vi "Calibration.vi"(8 "error in (no error)":errorcluster, 11 "VISA resource name In":T1={"Conection Data"="COM4"}) -> (0 "error out":errorcluster, 3 "VISA resource name Out":T1={"Conection Data"="COM4"})   [LabVIEW 2014, in "AD4212C Lib.lvlib"]
doc: "VI de calibración que se utiliza para poner a punto la balanza."
uses:
  AD4212C Lib.lvlib
  Typedef/Connection Data.ctl
  Typedef/Calibration Enum.ctl
panel:
  out "Indicator Med":string
  in  "Stop":bool
  out "Progress Bar":u64(slide) scale=0.0..6.0
  out "Indicator":string
  in  "Next":bool
  in  "Start":bool
  # "BALANCE CALIBRATION"
  # "Progress Bar"
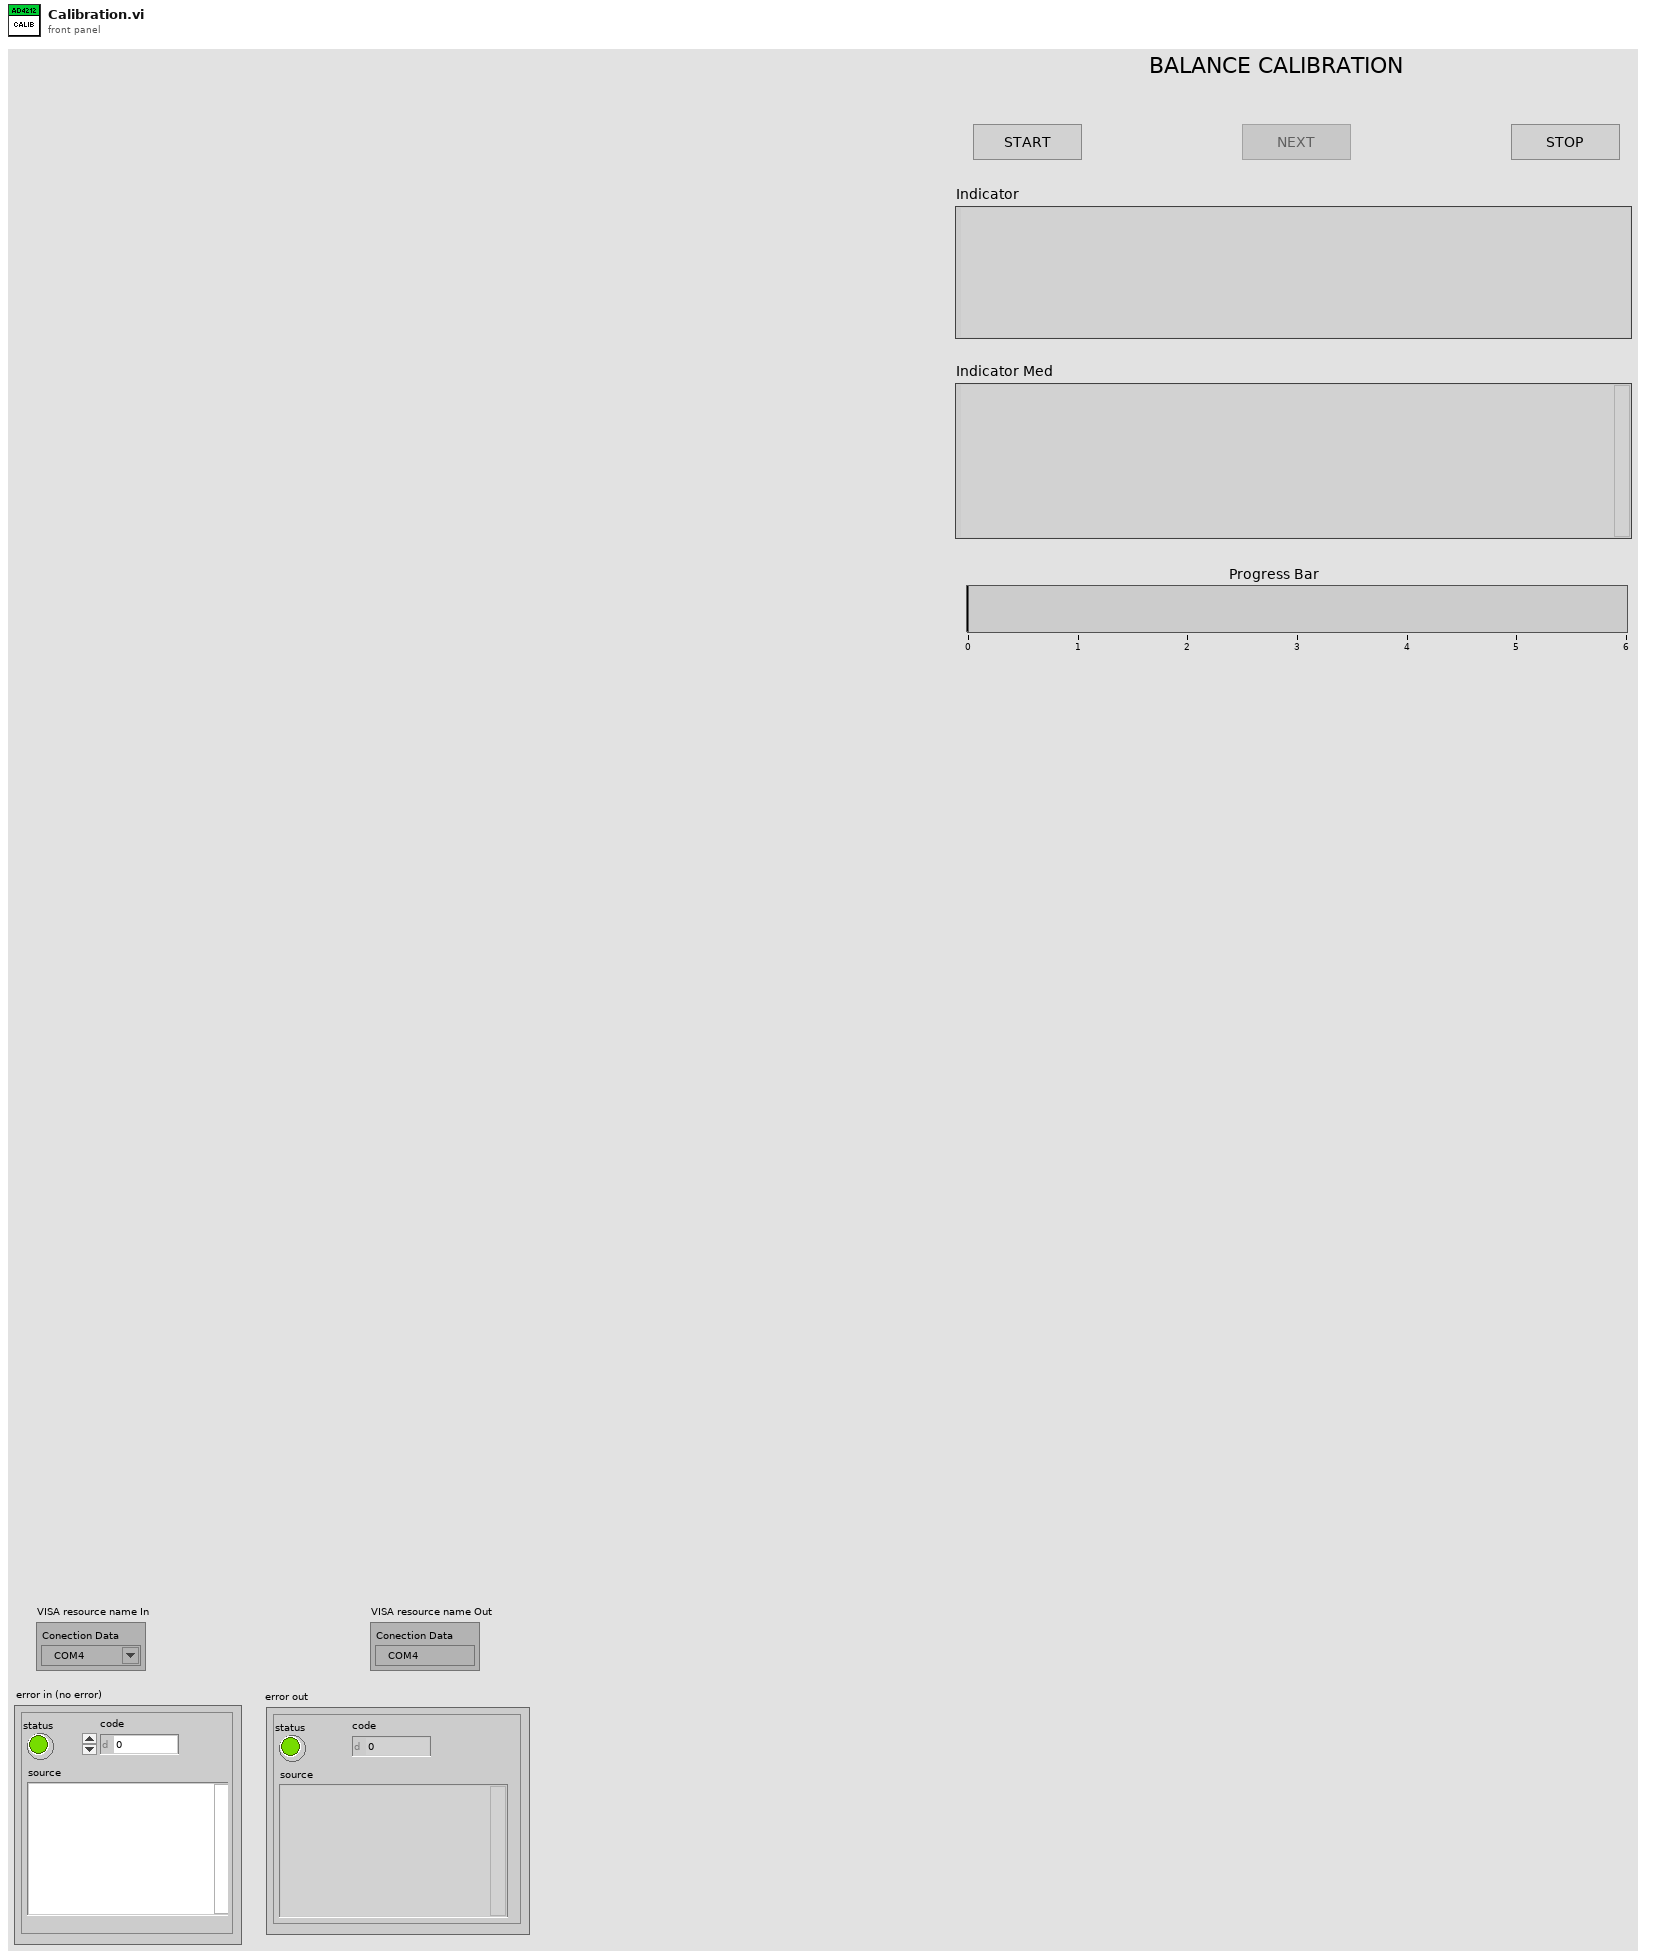
[diagram p1: front panel]
types:
  T1 = typedef "AD4212C Lib.lvlib/Connection Data.ctl" = cluster{"Conection Data":refnum<visa-resource-name>}
  T2 = typedef "AD4212C Lib.lvlib/Calibration Enum.ctl" = enum16{"Init", "Connection Open", "Start Calibration", "Idle Start", "Calibration Get Current Status 1", "Idle1 Next", "Calibration Get Current Status 2", "Idle2 Next", "Wait & Insert", "Calibration Get Current Status 3", "Idle3 Next", "Connection Close", "Idle Final"}
  T3 = enum8{"Enabled", "Disabled", "Disabled and Grayed Out"}
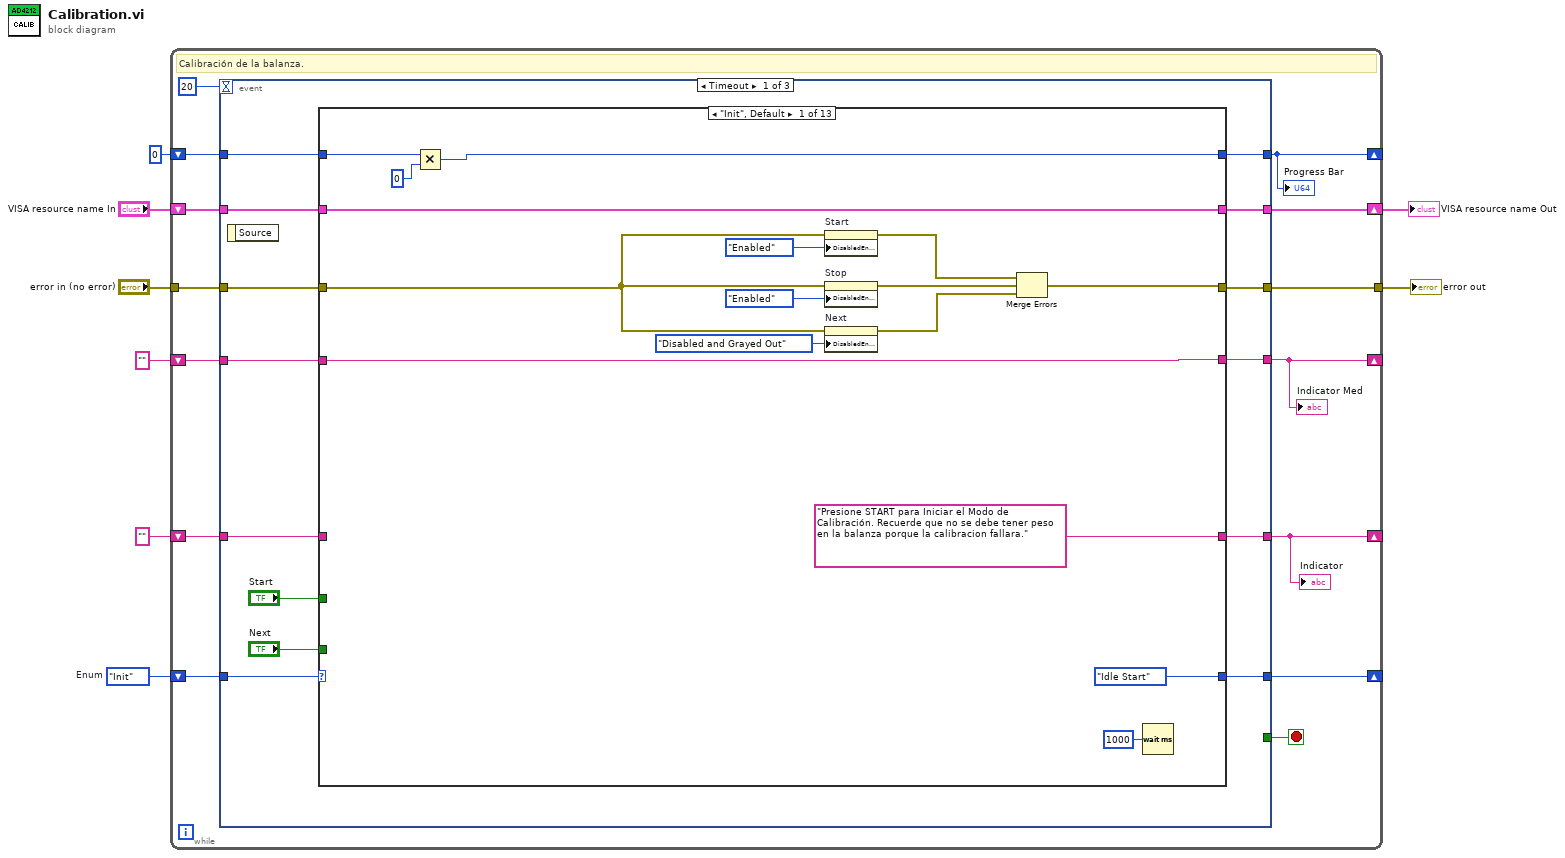
[diagram p0: block diagram]
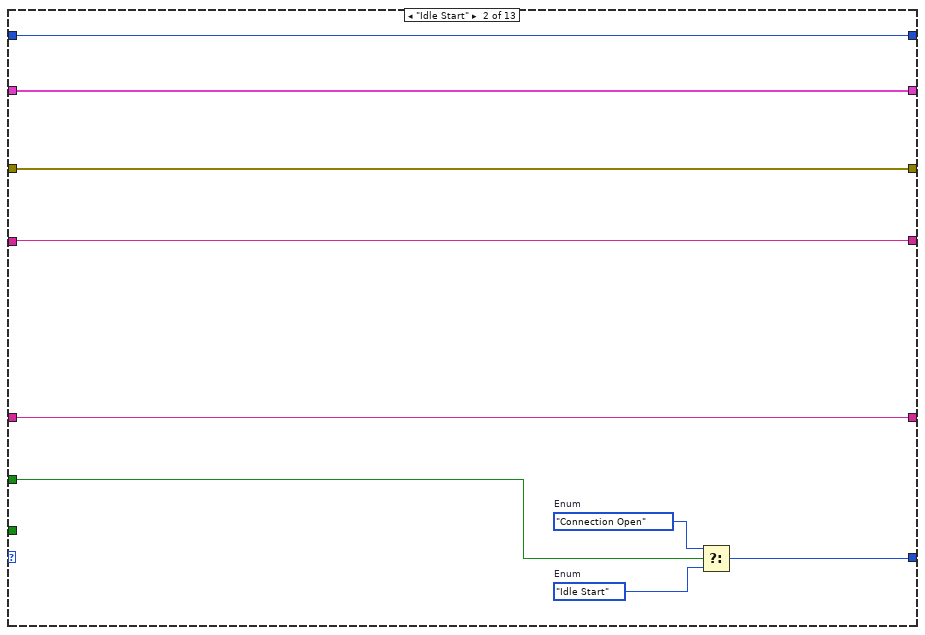
[diagram p2: hidden frame]
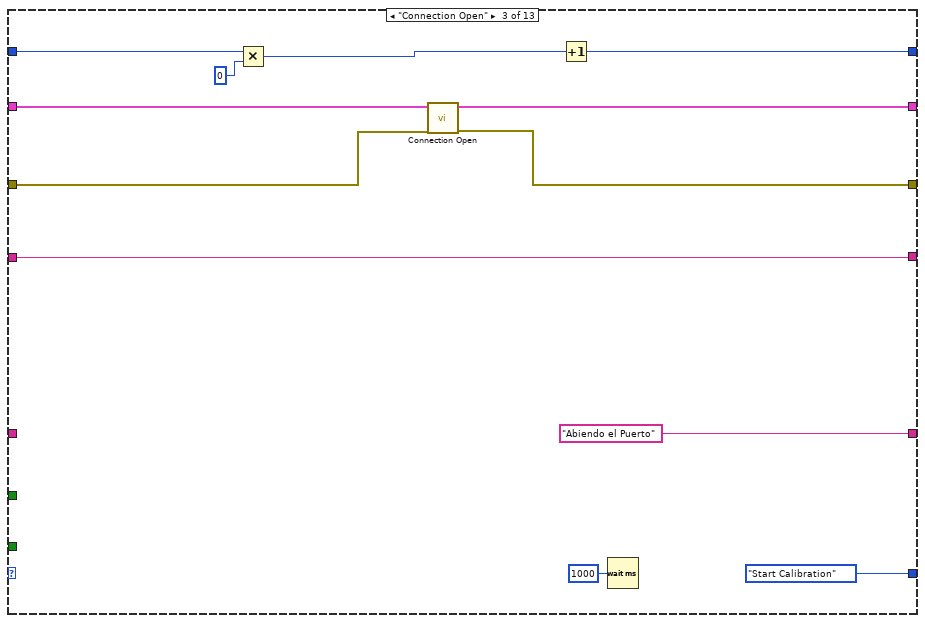
[diagram p3: hidden frame]
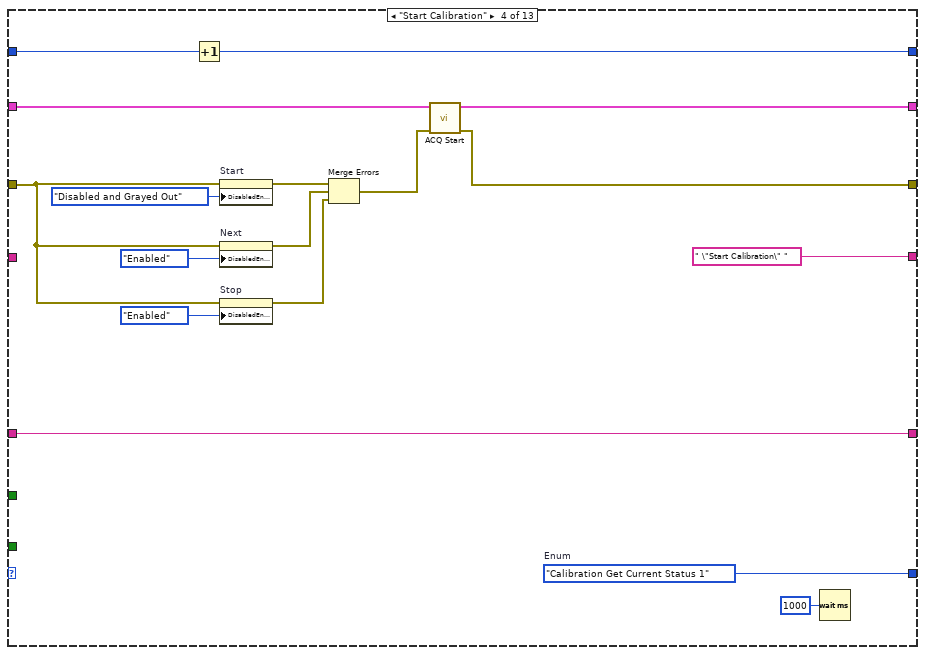
[diagram p4: hidden frame]
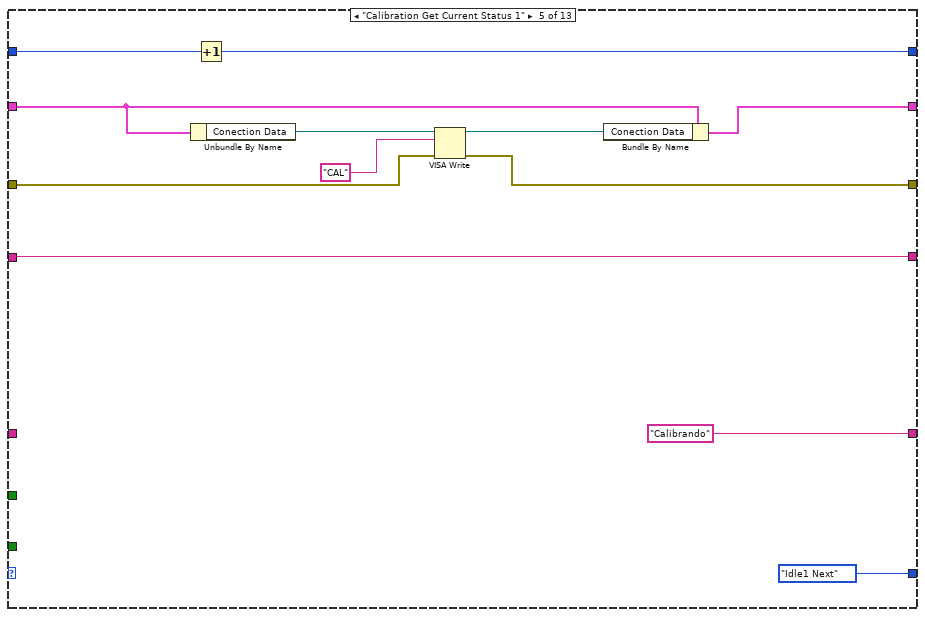
[diagram p5: hidden frame]
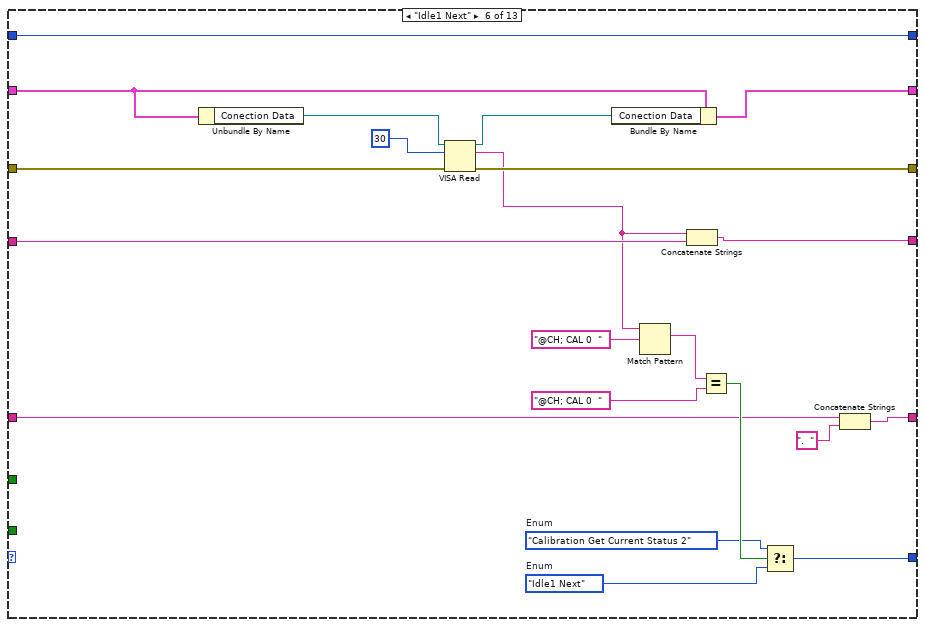
[diagram p6: hidden frame]
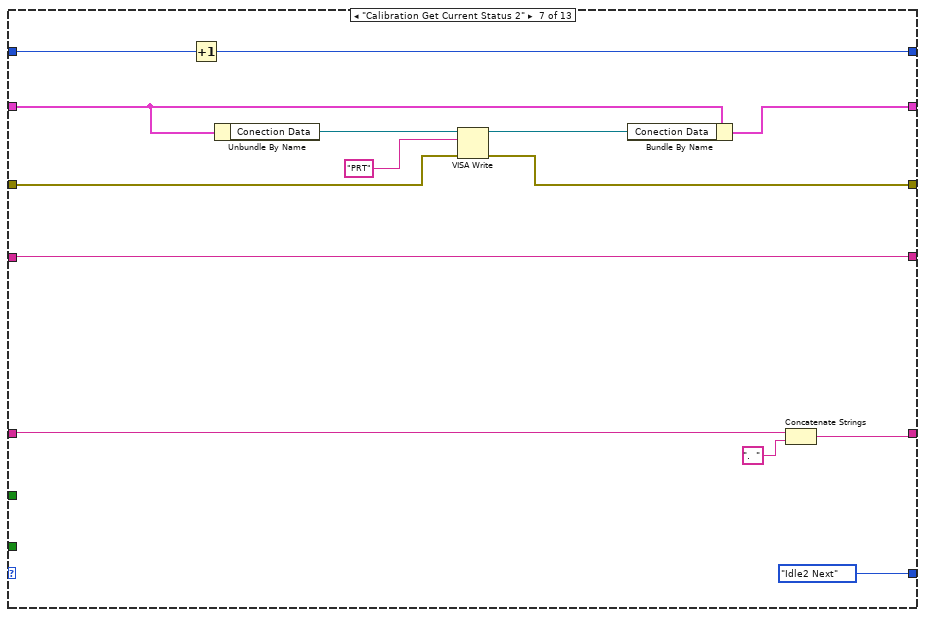
[diagram p7: hidden frame]
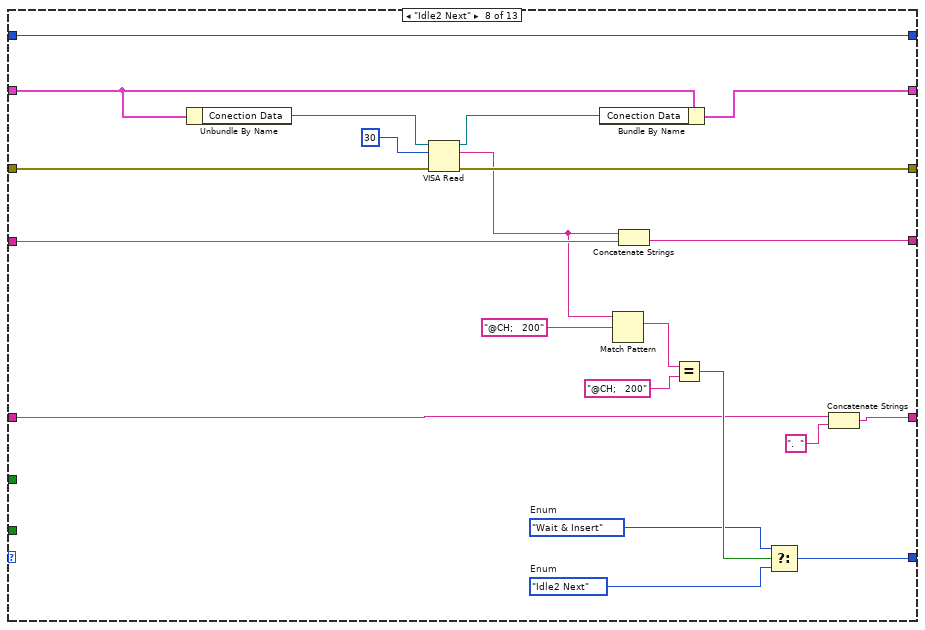
[diagram p8: hidden frame]
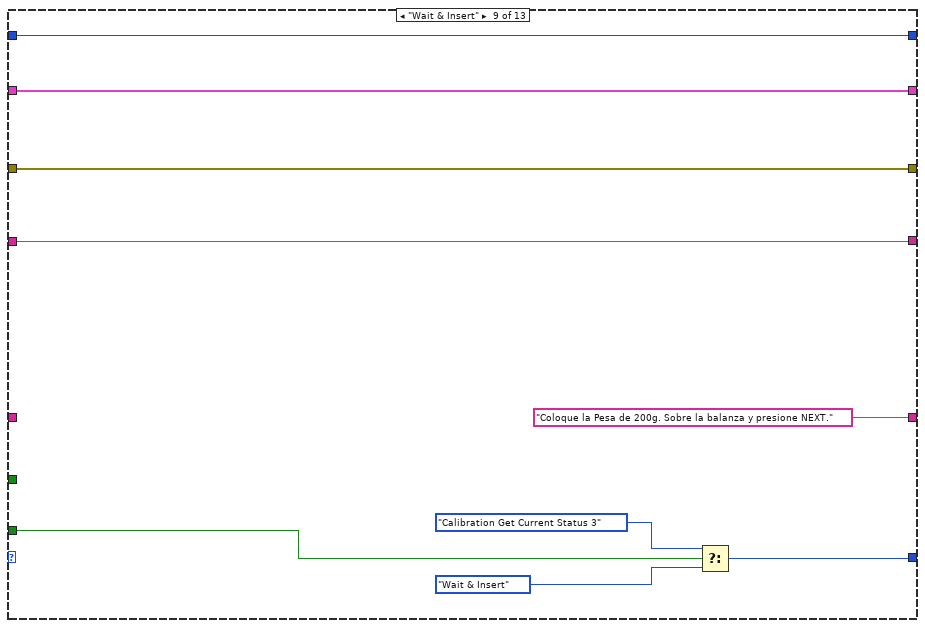
[diagram p9: hidden frame]
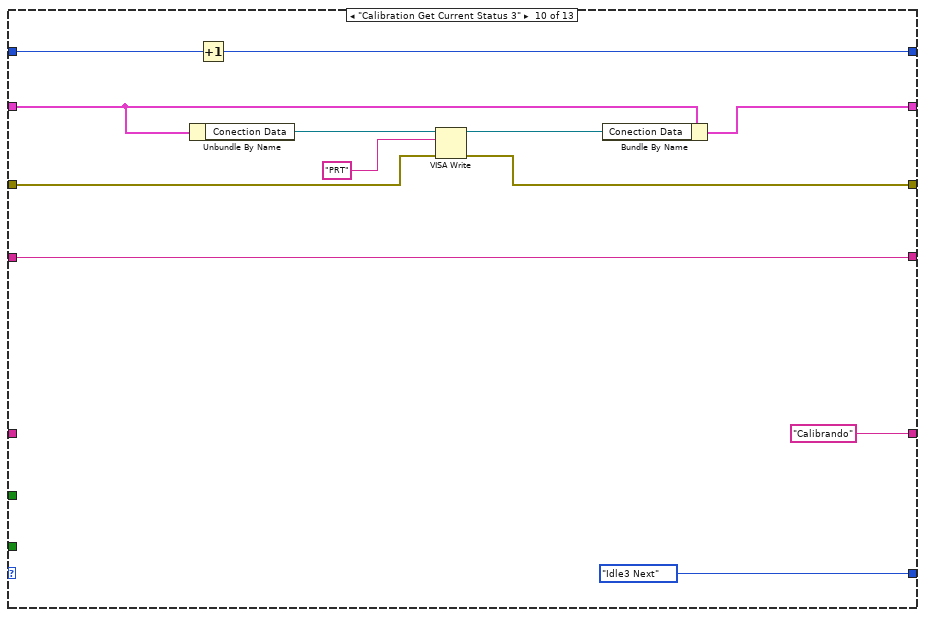
[diagram p10: hidden frame]
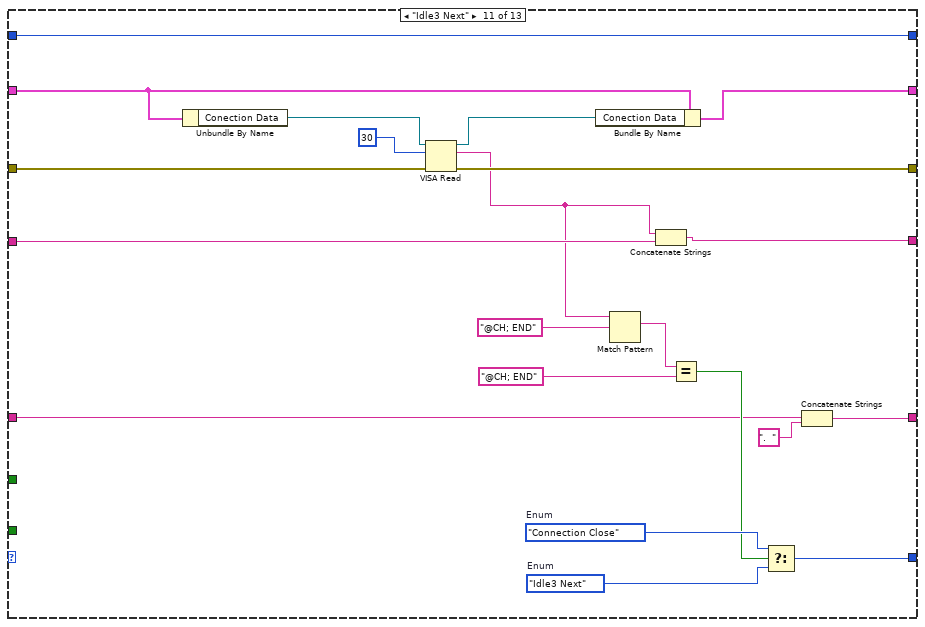
[diagram p11: hidden frame]
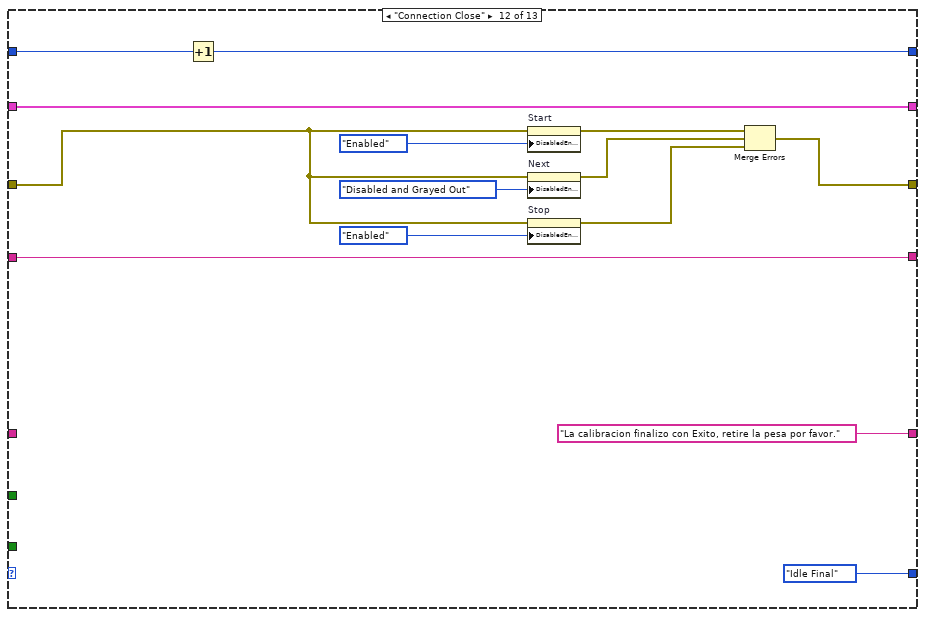
[diagram p12: hidden frame]
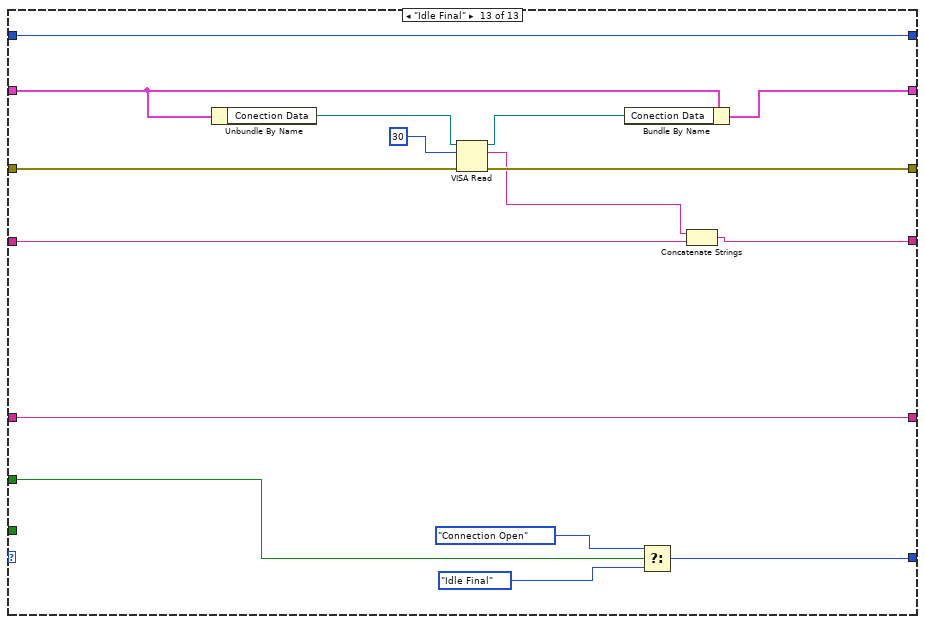
[diagram p13: hidden frame]
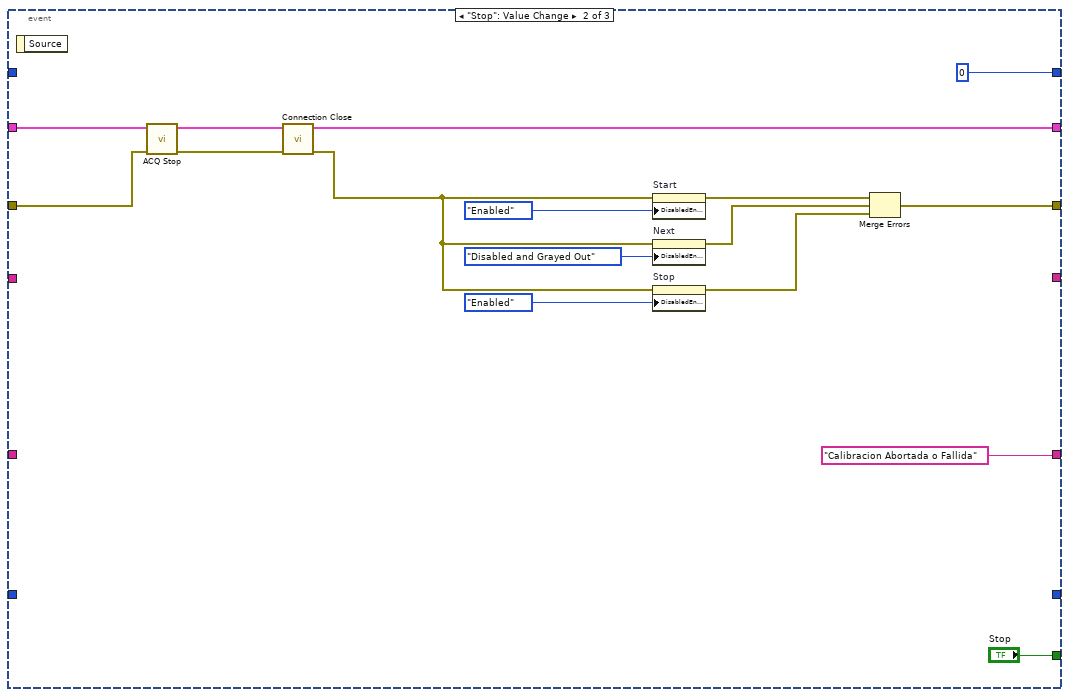
[diagram p14: hidden frame]
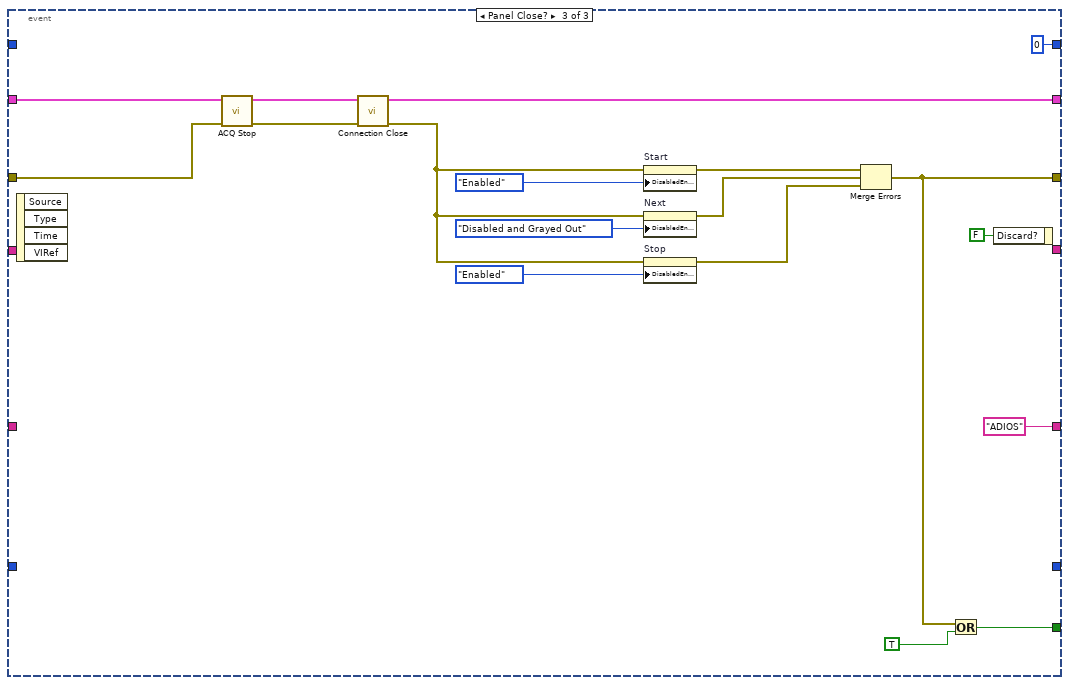
[diagram p15: hidden frame]
diagram:
  w1 = Calibration_Enum."Init"  # Enum
  n1 = while {
    tunnel: [w20] -> w7
    shift-right: [w16] -> w8
    shift-left: "VISA resource name In" -> [w22]
    shift-right: [w14] -> _
    shift-left: u64 0 ("Progress Status") -> [w19]
    shift-right: [w15] -> _
    shift-left: "" ("Caption.Text") -> [w17]
    tunnel: "error in (no error)" -> [w13]
    shift-right: [w12] -> _
    shift-left: "" ("read buffer") -> [w11]
    shift-right: [w9] -> _
    shift-left: w1 -> [w10]
    stop <- w21 stop-if-true
    # "Calibración de la balanza."
    n2 = event shown="[0] Timeout" {
      selector: _ -> [_ _ _]
      dyn-events: _ -> [_ _ _]
      timeout: 20 -> [_ _ _]
      tunnel: w22 -> [w36 w242 w259]
      tunnel: [_ "Stop" w262] -> w21
      tunnel: [w35 w231 w247] -> w20
      tunnel: w19 -> [w34 _ _]
      tunnel: [w33 u64 0 ("Progress Status") u64 0 ("Progress Status")] -> w14
      tunnel: [w32 "Calibracion Abortada o Fallida" ("Caption.Text") "ADIOS" ("Caption.Text")] -> w15
      tunnel: w17 -> [w31 _ _]
      tunnel: [w30 w241 w257] -> w16
      tunnel: w13 -> [w29 w240 w256]
      tunnel: [w26 _ _] -> w12
      tunnel: w11 -> [w25 _ _]
      tunnel: w10 -> [w24 _ _]
      tunnel: [w23 _ _] -> w9
      event Timeout {
        n3 = event-data() -> ()  [unwired: 1 in, 1 out]
        n4 = case shown="\"Init\", Default" w24 {
          tunnel: w36 -> [w43 w55 w71 w88 w91 w104 w127 w138 w163 w171 w180 w202 w215]
          tunnel: [w40 w56 w68 w86 w99 w123 w136 w158 w162 w178 w196 w207 w223] -> w35
          tunnel: ["Presione START para Iniciar el Modo de Calibración. Recuerde que no se debe tener peso en la balanza porque la calibracion fallara." ("Indicator") w60 "Abiendo el Puerto" ("Indicator") w89 "Calibrando" ("f") w109 w129 w143 "Coloque la Pesa de 200g. Sobre la balanza y presione NEXT." ("Caption.Text") "Calibrando" ("Caption.Text") w185 "La calibracion finalizo con Exito, retire la pesa por favor." ("Caption.Text") w219] -> w32
          tunnel: [w38 w61 w72 w75 w101 w110 w132 w145 w159 w173 w187 w203 w226] -> w33
          tunnel: w34 -> [w39 w61 w63 w76 w102 w110 w133 w145 w159 w174 w187 w204 w226]
          tunnel: w31 -> [_ w60 _ w89 _ w107 w128 w142 _ _ w184 _ w219]
          tunnel: [w43 w55 w70 w87 w92 w103 w126 w141 w163 w170 w183 w202 w216] -> w30
          tunnel: w29 -> [w44 w56 w69 w78 w98 w112 w135 w148 w162 w177 w189 w201 w224]
          tunnel: "Start" -> [_ w59 _ _ _ _ _ _ _ _ _ _ w230]
          tunnel: "Next" -> [_ _ _ _ _ _ _ _ w165 _ _ _ _]
          tunnel: [w41 w53 w65 " \"Start Calibration\" " ("read buffer") w95 w114 w134 w149 w161 w175 w191 w206 w222] -> w26
          tunnel: w25 -> [w41 w53 w65 _ w95 w116 w134 w151 w161 w175 w193 w206 w221]
          tunnel: [Calibration_Enum."Idle Start" ("Enum") w54 Calibration_Enum."Start Calibration" ("Enum") w74 Calibration_Enum."Idle1 Next" ("Enum") w111 Calibration_Enum."Idle2 Next" ("Enum") w147 w164 Calibration_Enum."Idle3 Next" ("Enum") w188 Calibration_Enum."Idle Final" ("Enum") w227] -> w23
          frame "Init", Default {
            n5 = Multiply(x=w39, y=u64 0) -> (x*y=w38:u64)
            n6 = property on="Start" class="Bool"(error in=w44, "DisabledEnum"=T3."Enabled" ("Disabled")) -> (error out=w50:errorcluster)  [unwired: 1 in, 1 out]
            n7 = property on="Stop" class="Bool"(error in=w44, "DisabledEnum"=T3."Enabled" ("Disabled")) -> (error out=w49:errorcluster)  [unwired: 1 in, 1 out]
            n8 = property on="Next" class="Bool"(error in=w44, "DisabledEnum"=T3."Disabled and Grayed Out" ("Disabled")) -> (error out=w48:errorcluster)  [unwired: 1 in, 1 out]
            n9 = Merge Errors(w50, w49, w48) -> (w40:errorcluster)
            n10 = Wait (ms)(milliseconds to wait=u32 1000) -> ()  [unwired: 1 out]
          }
          frame "Idle Start" {
            w57 = Calibration_Enum."Connection Open"  # Enum
            w58 = Calibration_Enum."Idle Start"  # Enum
            n11 = Select(t=w57, s=w59, f=w58) -> (s? t:f=w54:T2)
          }
          frame "Connection Open" {
            n12 = Multiply(x=w63, y=u64 0) -> (x*y=w62:u64)
            n13 = call "Connection Open.vi"("VISA resource name Out 3"=w71, "error in (no error)"=w69) -> ("VISA resource name Out 2"=w70:T1, "error out"=w68:errorcluster)  [unwired: 7 in]
            n14 = Increment(x=w62) -> (x+1=w72:u64)
            n15 = Wait (ms)(milliseconds to wait=u32 1000) -> ()  [unwired: 1 out]
          }
          frame "Start Calibration" {
            w74 = Calibration_Enum."Calibration Get Current Status 1"  # Enum
            n16 = Increment(x=w76) -> (x+1=w75:u64)
            n17 = property on="Start" class="Bool"(error in=w78, "DisabledEnum"=T3."Disabled and Grayed Out" ("Disabled")) -> (error out=w81:errorcluster)  [unwired: 1 in, 1 out]
            n18 = property on="Next" class="Bool"(error in=w78, "DisabledEnum"=T3."Enabled" ("Disabled")) -> (error out=w80:errorcluster)  [unwired: 1 in, 1 out]
            n19 = property on="Stop" class="Bool"(error in=w78, "DisabledEnum"=T3."Enabled" ("Disabled")) -> (error out=w79:errorcluster)  [unwired: 1 in, 1 out]
            n20 = Merge Errors(w81, w80, w79) -> (w82:errorcluster)
            n21 = call "ACQ Start.vi"("error in (no error)"=w82, "VISA resource name In"=w88) -> ("error out"=w86:errorcluster, "VISA resource name Out"=w87:T1)  [unwired: 8 in]
            n22 = Wait (ms)(milliseconds to wait=u32 1000) -> ()  [unwired: 1 out]
          }
          frame "Calibration Get Current Status 1" {
            n23 = Unbundle By Name(w91) -> ("Conection Data"=w94:refnum<visa-resource-name>)
            n24 = Increment(x=w102) -> (x+1=w101:u64)
            n25 = VISA Write(VISA resource name=w94, write buffer="CAL", error in (no error)=w98) -> (VISA resource name out=w93:refnum<visa-resource-name>, error out=w99:errorcluster)  [unwired: 1 out]
            n26 = Bundle By Name(cluster=w91, "Conection Data"=w93) -> (w92:T1)
          }
          frame "Idle1 Next" {
            w117 = Calibration_Enum."Idle1 Next"  # Enum
            w118 = Calibration_Enum."Calibration Get Current Status 2"  # Enum
            n27 = Unbundle By Name(w104) -> ("Conection Data"=w105:refnum<visa-resource-name>)
            n28 = VISA Read(VISA resource name=w105, byte count=u32 30 ("バイトカウント（0）"), error in (no error)=w112) -> (VISA resource name out=w106:refnum<visa-resource-name>, read buffer=w115:string, error out=w123:errorcluster)  [unwired: 1 out]
            n29 = Bundle By Name(cluster=w104, "Conection Data"=w106) -> (w103:T1)
            n30 = Match Pattern(string=w115, regular expression="@CH; CAL 0  ") -> (match substring=w121:string)  [unwired: 1 in, 3 out]
            n31 = Concatenate Strings(w115, w116) -> (w114:string)
            n32 = Equal?(x=w121, y="@CH; CAL 0  ") -> (x = y?=w119:bool)
            n33 = Select(t=w118, s=w119, f=w117) -> (s? t:f=w111:T2)
            n34 = Concatenate Strings(w107, ".  " ("string")) -> (w109:string)
          }
          frame "Calibration Get Current Status 2" {
            n35 = Increment(x=w133) -> (x+1=w132:u64)
            n36 = Unbundle By Name(w127) -> ("Conection Data"=w124:refnum<visa-resource-name>)
            n37 = VISA Write(VISA resource name=w124, write buffer="PRT", error in (no error)=w135) -> (VISA resource name out=w125:refnum<visa-resource-name>, error out=w136:errorcluster)  [unwired: 1 out]
            n38 = Bundle By Name(cluster=w127, "Conection Data"=w125) -> (w126:T1)
            n39 = Concatenate Strings(w128, ".  " ("string")) -> (w129:string)
          }
          frame "Idle2 Next" {
            w146 = Calibration_Enum."Wait & Insert"  # Enum
            w154 = Calibration_Enum."Idle2 Next"  # Enum
            n40 = Unbundle By Name(w138) -> ("Conection Data"=w139:refnum<visa-resource-name>)
            n41 = VISA Read(VISA resource name=w139, byte count=u32 30 ("バイトカウント（0）"), error in (no error)=w148) -> (VISA resource name out=w140:refnum<visa-resource-name>, read buffer=w150:string, error out=w158:errorcluster)  [unwired: 1 out]
            n42 = Bundle By Name(cluster=w138, "Conection Data"=w140) -> (w141:T1)
            n43 = Match Pattern(string=w150, regular expression="@CH;   200") -> (match substring=w156:string)  [unwired: 1 in, 3 out]
            n44 = Concatenate Strings(w150, w151) -> (w149:string)
            n45 = Equal?(x=w156, y="@CH;   200") -> (x = y?=w153:bool)
            n46 = Select(t=w146, s=w153, f=w154) -> (s? t:f=w147:T2)
            n47 = Concatenate Strings(w142, ".  " ("string")) -> (w143:string)
          }
          frame "Wait & Insert" {
            n48 = Select(t=Calibration_Enum."Calibration Get Current Status 3" ("Enum"), s=w165, f=Calibration_Enum."Wait & Insert" ("Enum")) -> (s? t:f=w164:T2)
          }
          frame "Calibration Get Current Status 3" {
            n49 = Unbundle By Name(w171) -> ("Conection Data"=w168:refnum<visa-resource-name>)
            n50 = Increment(x=w174) -> (x+1=w173:u64)
            n51 = VISA Write(VISA resource name=w168, write buffer="PRT", error in (no error)=w177) -> (VISA resource name out=w169:refnum<visa-resource-name>, error out=w178:errorcluster)  [unwired: 1 out]
            n52 = Bundle By Name(cluster=w171, "Conection Data"=w169) -> (w170:T1)
          }
          frame "Idle3 Next" {
            w198 = Calibration_Enum."Idle3 Next"  # Enum
            w199 = Calibration_Enum."Connection Close"  # Enum
            n53 = Unbundle By Name(w180) -> ("Conection Data"=w181:refnum<visa-resource-name>)
            n54 = VISA Read(VISA resource name=w181, byte count=u32 30 ("バイトカウント（0）"), error in (no error)=w189) -> (VISA resource name out=w182:refnum<visa-resource-name>, read buffer=w192:string, error out=w196:errorcluster)  [unwired: 1 out]
            n55 = Bundle By Name(cluster=w180, "Conection Data"=w182) -> (w183:T1)
            n56 = Match Pattern(string=w192, regular expression="@CH; END" ("y")) -> (match substring=w200:string)  [unwired: 1 in, 3 out]
            n57 = Concatenate Strings(w192, w193) -> (w191:string)
            n58 = Equal?(x=w200, y="@CH; END") -> (x = y?=w197:bool)
            n59 = Select(t=w199, s=w197, f=w198) -> (s? t:f=w188:T2)
            n60 = Concatenate Strings(w184, ".  " ("string")) -> (w185:string)
          }
          frame "Connection Close" {
            n61 = Increment(x=w204) -> (x+1=w203:u64)
            n62 = property on="Start" class="Bool"(error in=w201, "DisabledEnum"=T3."Enabled" ("Disabled")) -> (error out=w213:errorcluster)  [unwired: 1 in, 1 out]
            n63 = property on="Next" class="Bool"(error in=w201, "DisabledEnum"=T3."Disabled and Grayed Out" ("Disabled")) -> (error out=w212:errorcluster)  [unwired: 1 in, 1 out]
            n64 = property on="Stop" class="Bool"(error in=w201, "DisabledEnum"=T3."Enabled" ("Disabled")) -> (error out=w211:errorcluster)  [unwired: 1 in, 1 out]
            n65 = Merge Errors(w213, w212, w211) -> (w207:errorcluster)
          }
          frame "Idle Final" {
            n66 = Unbundle By Name(w215) -> ("Conection Data"=w217:refnum<visa-resource-name>)
            n67 = VISA Read(VISA resource name=w217, byte count=u32 30 ("バイトカウント（0）"), error in (no error)=w224) -> (VISA resource name out=w218:refnum<visa-resource-name>, read buffer=w220:string, error out=w223:errorcluster)  [unwired: 1 out]
            n68 = Bundle By Name(cluster=w215, "Conection Data"=w218) -> (w216:T1)
            n69 = Select(t=Calibration_Enum."Connection Open" ("Enum"), s=w230, f=Calibration_Enum."Idle Final" ("Enum")) -> (s? t:f=w227:T2)
            n70 = Concatenate Strings(w220, w221) -> (w222:string)
          }
        }
      }
      event "Stop": Value Change {
        n71 = event-data() -> ()  [unwired: 1 in, 1 out]
        n72 = call "ACQ Stop.vi"("error in (no error)"=w240, "VISA resource name In"=w242) -> ("error out"=w244:errorcluster, "VISA resource name Out"=w243:T1)  [unwired: 8 in]
        n73 = call "Connection Close.vi"("error in (no error)"=w244, "VISA resource name In"=w243) -> ("error out"=w232:errorcluster, "VISA resource name Out"=w241:T1)  [unwired: 8 in]
        n74 = property on="Start" class="Bool"(error in=w232, "DisabledEnum"=T3."Enabled" ("Disabled")) -> (error out=w238:errorcluster)  [unwired: 1 in, 1 out]
        n75 = property on="Next" class="Bool"(error in=w232, "DisabledEnum"=T3."Disabled and Grayed Out" ("Disabled")) -> (error out=w237:errorcluster)  [unwired: 1 in, 1 out]
        n76 = property on="Stop" class="Bool"(error in=w232, "DisabledEnum"=T3."Enabled" ("Disabled")) -> (error out=w236:errorcluster)  [unwired: 1 in, 1 out]
        n77 = Merge Errors(w238, w237, w236) -> (w231:errorcluster)
      }
      event Panel Close? {
        n78 = event-data() -> ()  [unwired: 1 in, 4 out]
        n79 = call "ACQ Stop.vi"("error in (no error)"=w256, "VISA resource name In"=w259) -> ("error out"=w255:errorcluster, "VISA resource name Out"=w258:T1)  [unwired: 8 in]
        n80 = call "Connection Close.vi"("error in (no error)"=w255, "VISA resource name In"=w258) -> ("error out"=w248:errorcluster, "VISA resource name Out"=w257:T1)  [unwired: 8 in]
        n81 = property on="Start" class="Bool"(error in=w248, "DisabledEnum"=T3."Enabled" ("Disabled")) -> (error out=w254:errorcluster)  [unwired: 1 in, 1 out]
        n82 = property on="Next" class="Bool"(error in=w248, "DisabledEnum"=T3."Disabled and Grayed Out" ("Disabled")) -> (error out=w253:errorcluster)  [unwired: 1 in, 1 out]
        n83 = property on="Stop" class="Bool"(error in=w248, "DisabledEnum"=T3."Enabled" ("Disabled")) -> (error out=w252:errorcluster)  [unwired: 1 in, 1 out]
        n84 = Merge Errors(w254, w253, w252) -> (w247:errorcluster)
        n85 = Or(x=w247, y=TRUE) -> (x .or. y?=w262:bool)
        n86 = event-data("Discard?"=FALSE) -> ()  [unwired: 1 in, 1 out]
      }
    }
    "Indicator" <- w15
    "Progress Bar" <- w14
    "Indicator Med" <- w12
  }
  "error out" <- w7
  "VISA resource name Out" <- w8
